vi "SpecAn Fetch IM.vi"(0 "RFmx Handle In":refnum<k21>, 1 "Selector String":string, 11 "error in (no error)":errorcluster) -> (4 "RFmx Handle Out":refnum<k21>, 6 "SpecAn IM Results":T1 {"Intermod Order Results"."Upper Intermod Power (dBm)" format="%.2f"; "Intermod Order Results"."Lower Intermod Power (dBm)" format="%.2f"; "Intermod Order Results"."Upper Output Intercept Power (dBm)" format="%.2f"; "Intermod Order Results"."Lower Output Intercept Power (dBm)" format="%.2f"; "Intermod Order Results"."Worst Case Output Intercept Power (dBm)" format="%.2f"; "Upper Tone Power (dBm)" format="%.2f"; "Lower Tone Power (dBm)" format="%.2f"}, 15 "error out":errorcluster)   [LabVIEW 2016, in "RFmxSpecAn.lvlib"]
doc: "Fetches common results from the IM measurement."
uses:
  RFmxSpecAn.lvlib
  Typedefs/SpecAn IM Results.ctl
  Typedefs/SpecAn IM Intermod Order Results.ctl
  <vilib>/RFmx/SpecAn/mx/RFmxSpecAn.llb/RFmxSpecAn IM Fetch Fundamental Measurement.vi
  <resource>/objmgr/RFmxSpecAn.rc
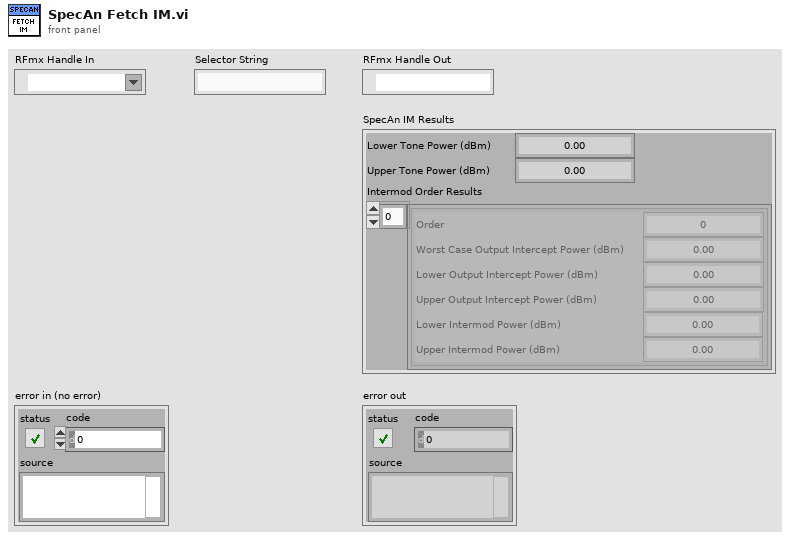
[diagram p1: front panel]
types:
  T1 = typedef "RFmxSpecAn.lvlib/SpecAn IM Results.ctl" = cluster{"Lower Tone Power (dBm)":dbl, "Upper Tone Power (dBm)":dbl, "Intermod Order Results":T2[]}
  T2 = typedef "RFmxSpecAn.lvlib/SpecAn IM Intermod Order Results.ctl" = cluster{"Order":i32, "Worst Case Output Intercept Power (dBm)":dbl, "Lower Output Intercept Power (dBm)":dbl, "Upper Output Intercept Power (dBm)":dbl, "Lower Intermod Power (dBm)":dbl, "Upper Intermod Power (dBm)":dbl}
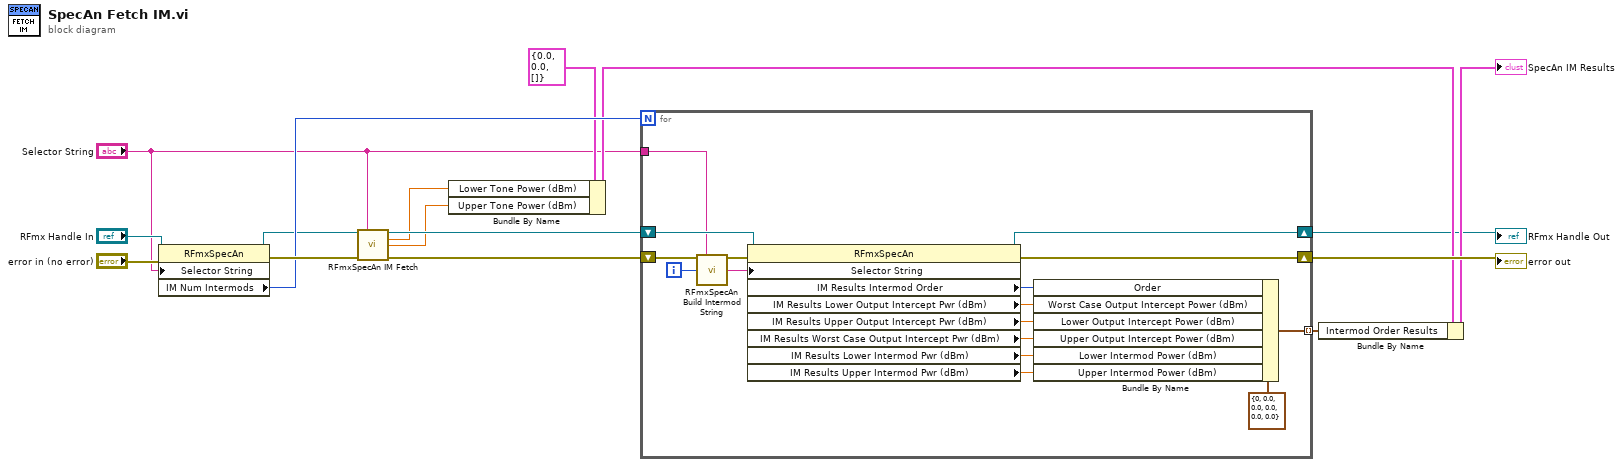
[diagram p0: block diagram]
diagram:
  n1 = property class="RFmxSpecAn"(reference="RFmx Handle In", error in="error in (no error)", "Selector String"="Selector String") -> (reference out=w6:refnum<k21>, error out=w15:errorcluster, "IM Num Intermods"=w11:i32)
  n2 = call-poly <vilib>:"RFmxSpecAn IM Fetch.vi"("Instrument Handle In"=w6, "Selector String"="Selector String", "error in (no error)"=w15) -> ("Instrument Handle Out"=w5:refnum<k21>, "Lower Tone Power (dBm)"=w4:dbl, "Upper Tone Power (dBm)"=w3:dbl, "error out"=w14:errorcluster)  [unwired: 9 in]
  n3 = Bundle By Name(cluster=T1 {"Lower Tone Power (dBm)"=0.0, "Upper Tone Power (dBm)"=0.0, "Intermod Order Results"=[]} ("SpecAn IM Results"), "Lower Tone Power (dBm)"=w4, "Upper Tone Power (dBm)"=w3) -> (w8:T1)
  n4 = for {
    N: w11 -> [_]
    shift-right: [w18] -> w1
    shift-left: w5 -> [w29]
    shift-right: [w31] -> w13
    shift-left: w14 -> [w30]
    tunnel: "Selector String" -> [w28]
    tunnel: [w17] -> w9 mode=indexing
    i -> [w27]
    n5 = call <vilib>:"RFmxSpecAn Build Intermod String.vi"("Selector String"=w28, "Intermod Number"=w27) -> ("Selector String Out"=w26:string)  [unwired: 13 in]
    n6 = property class="RFmxSpecAn"(reference=w29, error in=w30, "Selector String"=w26) -> (reference out=w18:refnum<k21>, error out=w31:errorcluster, "IM Results Intermod Order"=w24:i32, "IM Results Lower Output Intercept Pwr (dBm)"=w23:dbl, "IM Results Upper Output Intercept Pwr (dBm)"=w22:dbl, "IM Results Worst Case Output Intercept Pwr (dBm)"=w21:dbl, "IM Results Lower Intermod Pwr (dBm)"=w20:dbl, "IM Results Upper Intermod Pwr (dBm)"=w19:dbl)
    n7 = Bundle By Name(cluster=T2 {"Order"=0, "Worst Case Output Intercept Power (dBm)"=0.0, "Lower Output Intercept Power (dBm)"=0.0, "Upper Output Intercept Power (dBm)"=0.0, "Lower Intermod Power (dBm)"=0.0, "Upper Intermod Power (dBm)"=0.0} ("SpecAn IM Intermod Order Results"), "Order"=w24, "Worst Case Output Intercept Power (dBm)"=w23, "Lower Output Intercept Power (dBm)"=w22, "Upper Output Intercept Power (dBm)"=w21, "Lower Intermod Power (dBm)"=w20, "Upper Intermod Power (dBm)"=w19) -> (w17:T2)
  }
  "error out" <- w13
  "RFmx Handle Out" <- w1
  n8 = Bundle By Name(cluster=w8, "Intermod Order Results"=w9) -> (→"SpecAn IM Results":T1)
